vi "PPS Persistent TCP parser server.vi"(8 "error in":errorcluster, 9 "TCP queue name":string="parser_error", 10 "Ignore errors":bool=TRUE, 11 "port":u16=2056) -> (0 "error out":errorcluster)   [LabVIEW 2016]
uses:
  <vilib>/Utility/error.llb/DialogType.ctl
  <vilib>/Utility/error.llb/whitespace.ctl
panel:
  out "Listening":bool=TRUE
  out "Control labels":string
  out "Explanation":string
  out "created new?":bool
  out "TCP error queue":refnum<queue>
  out "cycle msec":u32
  out "Cmd Rec'd":bool
  out "Calling VI's Controls":string[](array[string])
  out "Idle loop":i32
  out "Heartbeat":bool=TRUE
  in  "bytes to read":i32=256
  out "ack":string
  in  "stop":bool=TRUE
  # "This subVI is currently written to handle controls of numeric (\"Digital\", \"Numeric\", \"Ring\"), string and boolean types, and queries of simple clusters and boolean & numeric arrays."
  # "# Example Python program\n\n# Drop this subVI into the VI you want to remote-enable.\n\n#  Here we assume the remote VI has an indicator named \"DisplayValue\" and a control named \"NumberControl\",\n#  and that an event is driven by a value change for NumberControl.\n\nimport os\nimport socket\nimport time\n\nTCP_IP = '127.0.0.1'  #...for VI running on same machine.  Else put IP address of remote machine.\nTCP_PORT = 2056  # Set the port in the VI that calls the parser server.  \nBUFFER_SIZE = 1024\n\n\n\ndef Transact(Command, IsAQuery):   \n\n    StuffToSend = Command + '\\r' + '\\n'   # The TCP Parser Server is looking for cr-lf termination\n    s.send(StuffToSend)\n    response = s.recv(BUFFER_SIZE)   # Communications is much more reliable if you read the response.  \n                                                               # Ideally, compare it to what you sent.  For simplicity we are not doing that here.\n\n    if IsAQuery:\n        response = response.translate(None,'\\r''\\n')  #remove terminator characters\n        return response\n\n#====== Here's the program =====\n\nprint 'Opening socket'\n\ns = socket.socket(socket.AF_INET, socket.SOCK_STREAM)\ns.setsockopt(socket.SOL_SOCKET, socket.SO_REUSEADDR, 1)\ns.connect((TCP_IP, TCP_PORT))\n\n\nfor i in range (1,5000):\n    QueryString = 'DisplayValue?'\n    CommandString = 'NumberControl=' + str(i)\n\n# Send a command\n    Transact (CommandString, False) # False indicates it is not a query\n\n# Perform a query and display the response\n    print 'Received:' + (Transact(QueryString, True)) # 'True' indicates it is a query\n    \n    \n    \ns.shutdown(socket.SHUT_RDWR)\ntime.sleep(0.02) # Delay to prevent a possible Windows error.  20msec is very generous.\ns.close()"
  # "This VI listens on the specified TCP port until a terminated command or query is seen.\n\n-- Command format: \"[Control name] = [new value] [CR][LF]\n\nThis VI will always echo the command it receives (after a CR/LF termination) in the ack indicator, also with CR/LF termination.  Good practice is to compare this return with the issued command to ensure against error.\n\n\n-- Query format: \"[Control or indicator name]?[CR][LF]\"  \n\nAfter query, the ack indicator will contain [Control or indicator name]=[value][CR][LF] \n\nWhite space in commands/queries is ignored.  Control names are case sensitive.\n\nSeparate array elements with tab characters, e.g.; NumberArray = 1\\t2\\t3\\t[CR][LF]\nSeparate cluster elements with vertical-bar characters, e.g.; error out|status?[CR][LF]"
  # "This parser can be made re-entrant to allow scripting of >1 top-level VIs.  The port is set by the calling VI,  take care not to duplicate.\n\nThe calling VI's front-panel controls are available in the indicator to the right.  Since this VI will not return until terminated, read the Calling VI's Controls indicator using a VI reference.  \n\nThe calling VI should have an Event Structure that fires on value change of the controls you want to remote-enable.   Currently supported types are Boolean, Digital (numeric) and String. \n\nAny front-panel control of a supported type can be queried.  \n\nThe instantaneous error status of this VI is available in a named queue.  The name is provided by the calling VI and must be unique.  (The name of the calling VI is a good choice.)"
  # "Note: we trap and internally handle error 66, which indicates a connection was closed.  \nWhen this occurs we simply re-open the connection.\nThis allows a remote host to run and finish many times."
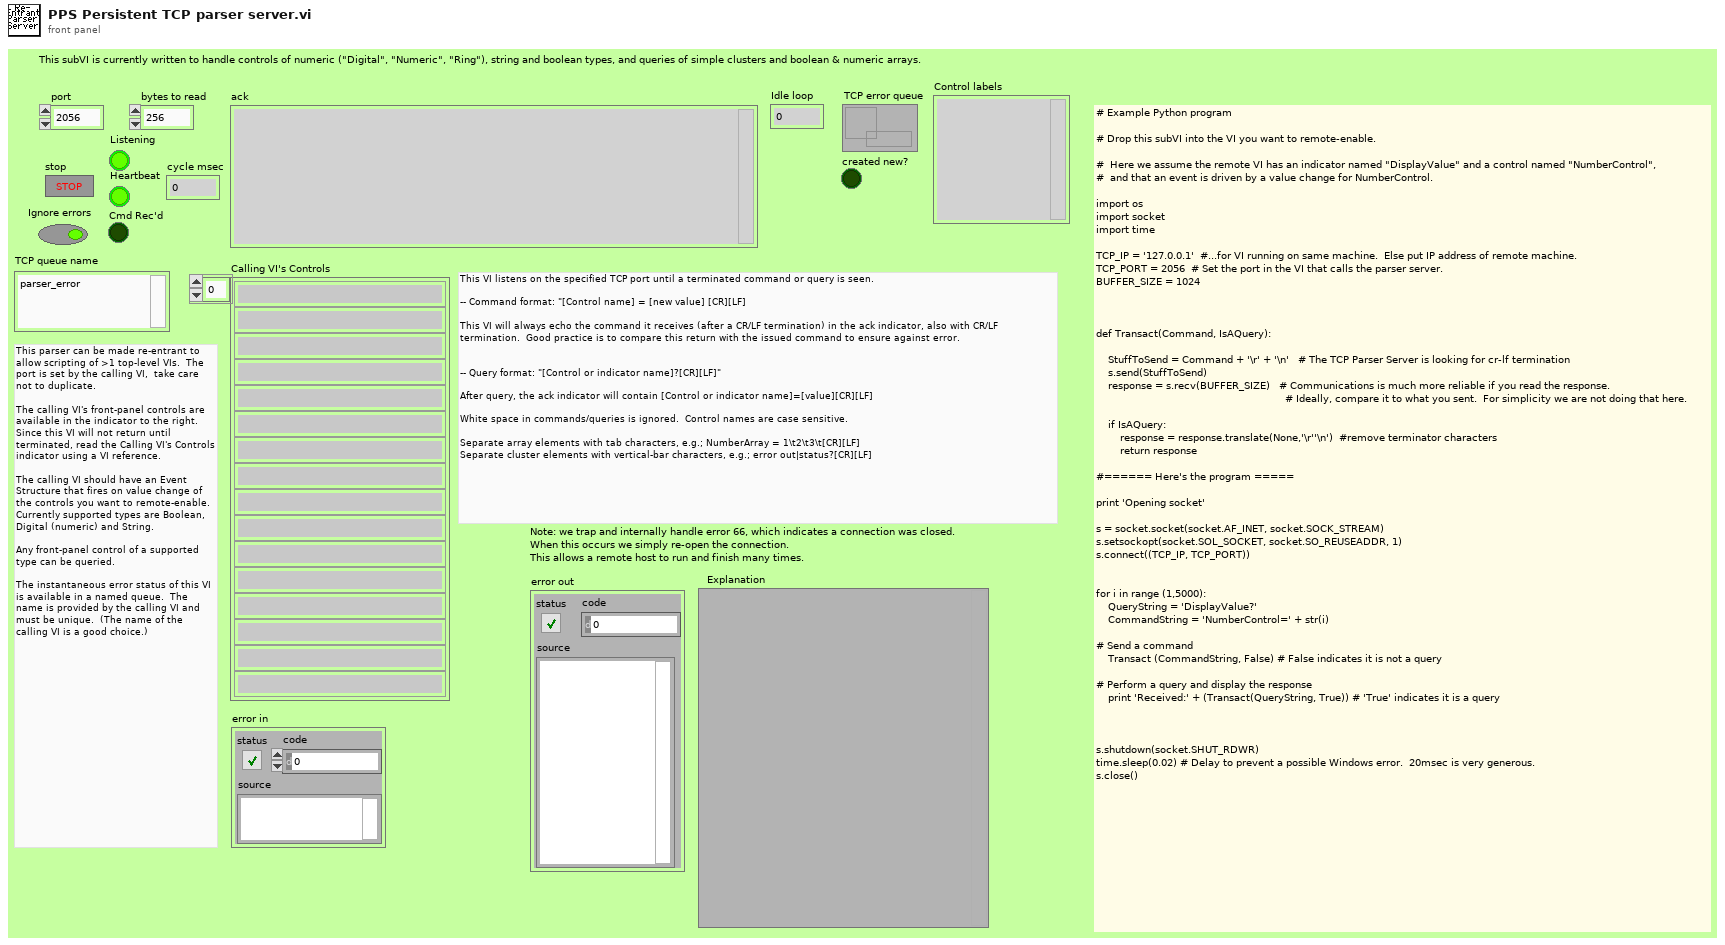
[diagram p1: front panel]
types:
  T1 = enum16{"Standard", "Buffered", "CRLF", "Immediate"}
  T2 = typedef "DialogType.ctl" = u16
  T3 = typedef "whitespace.ctl" = u16
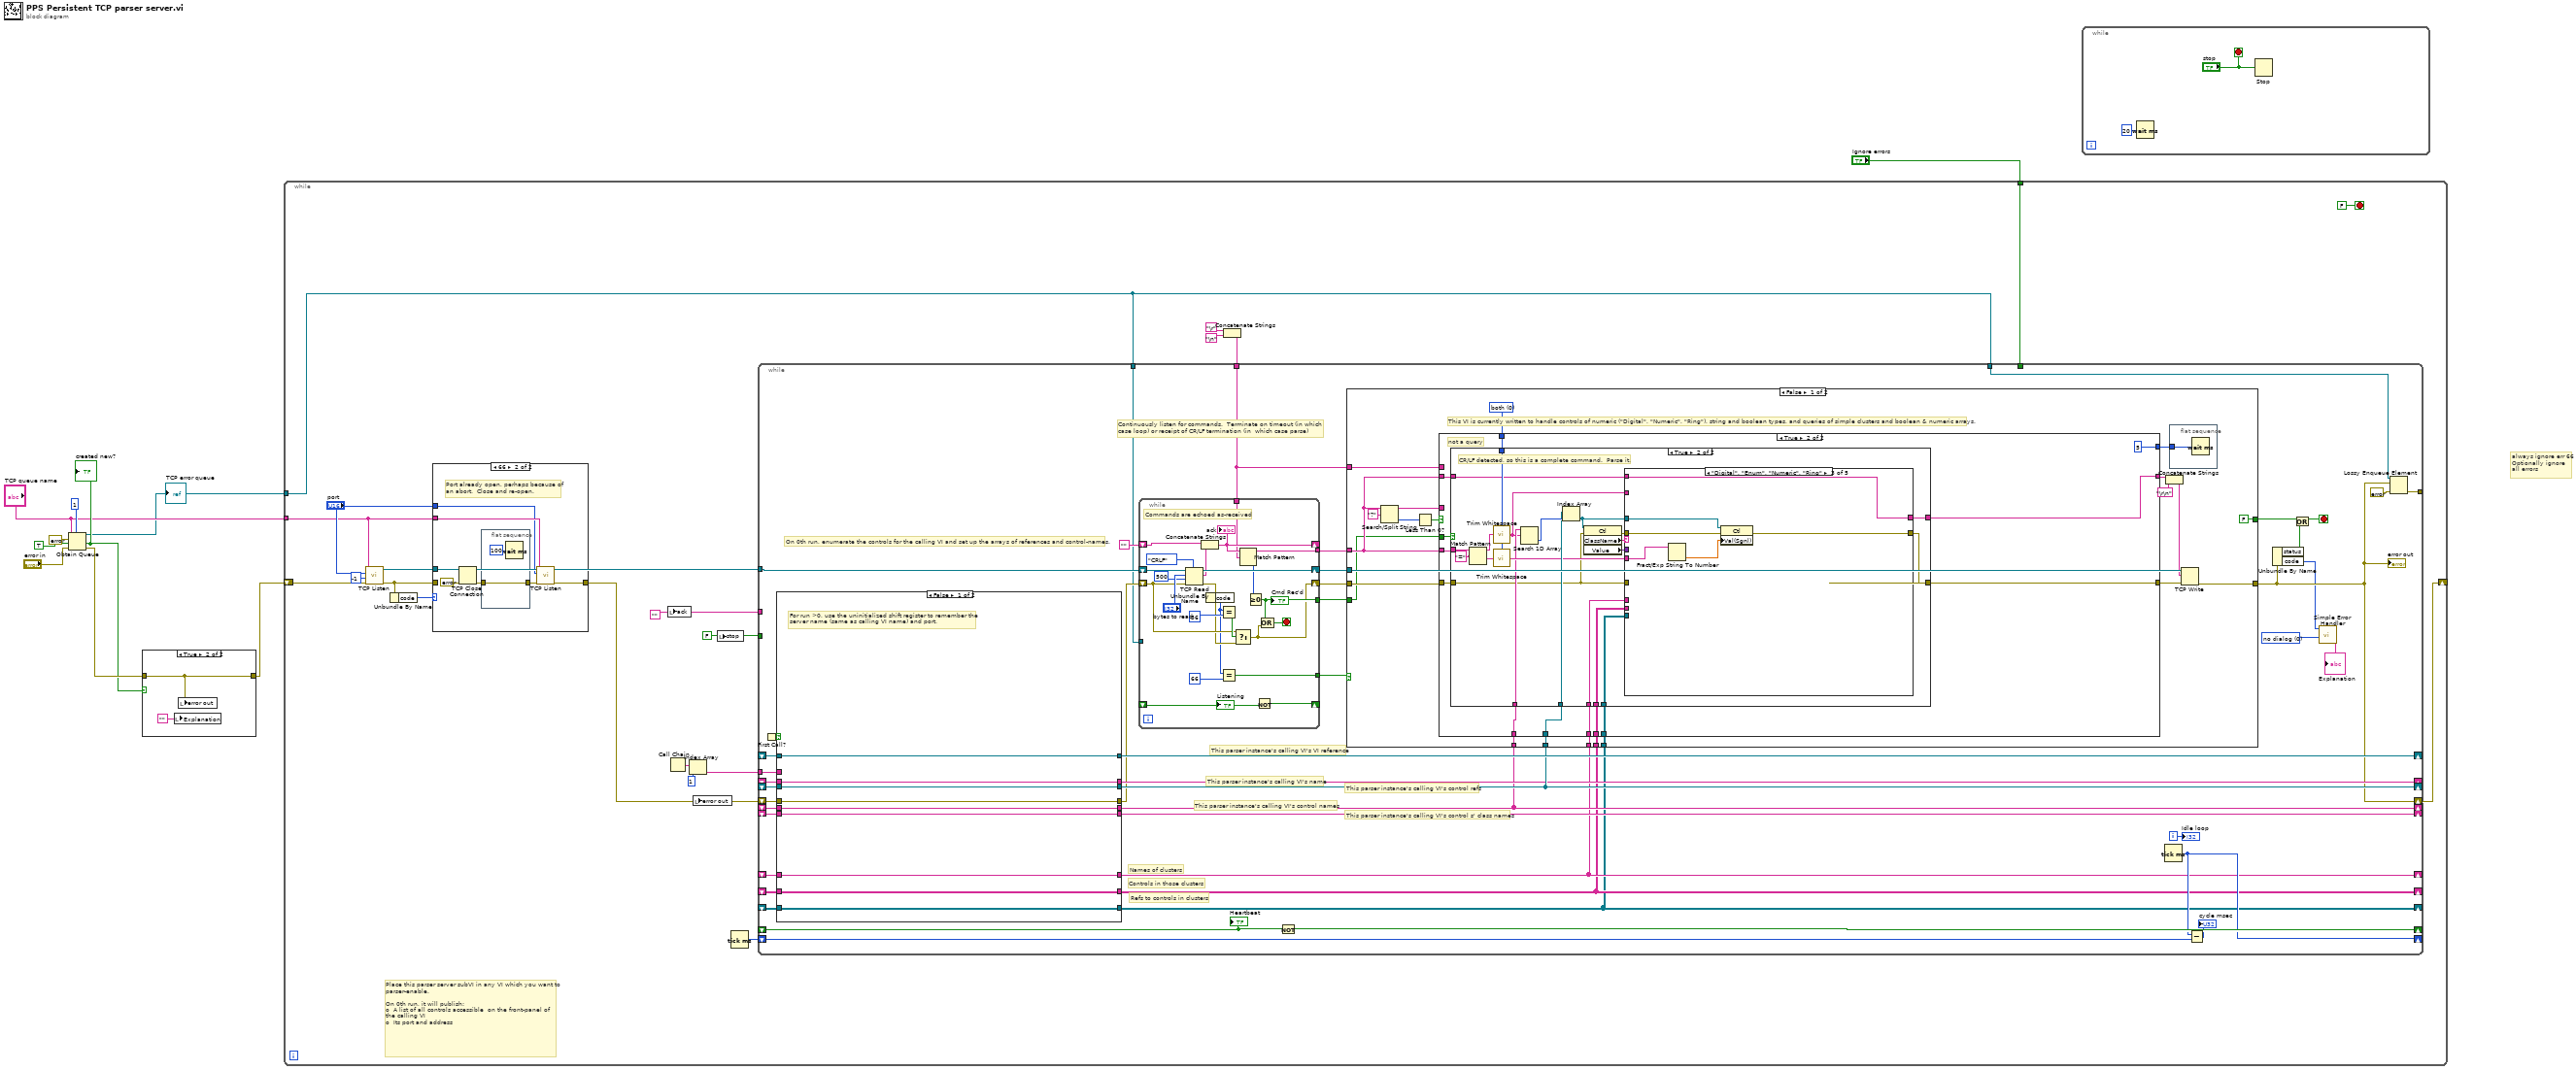
[diagram p0: block diagram]
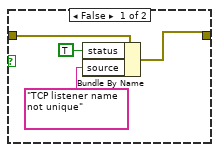
[diagram p2: hidden frame]
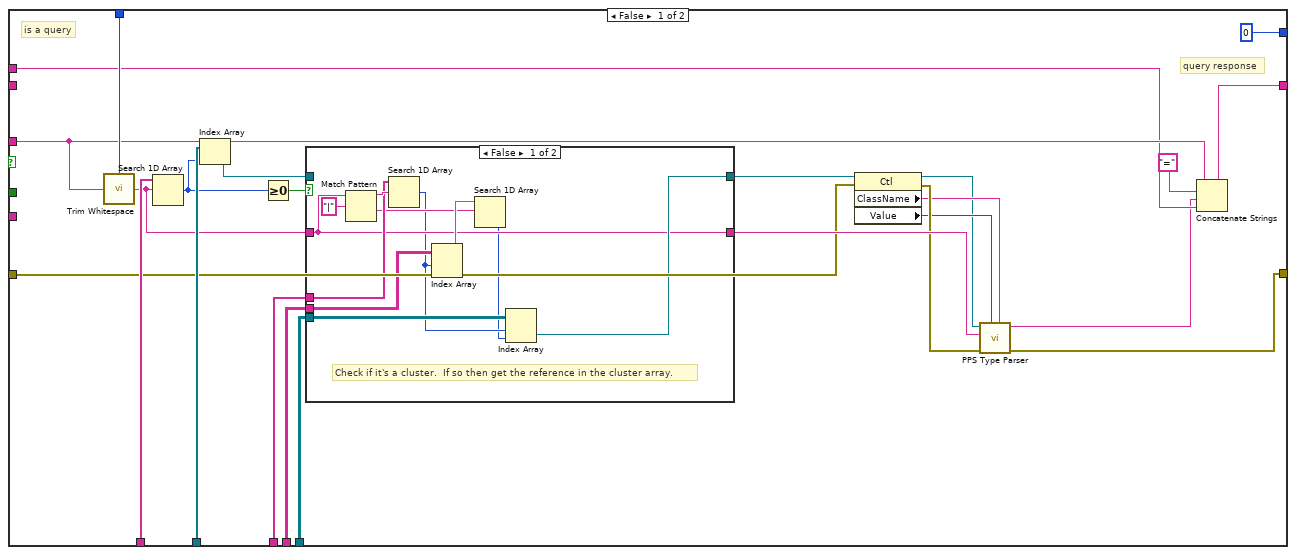
[diagram p4: hidden frame]
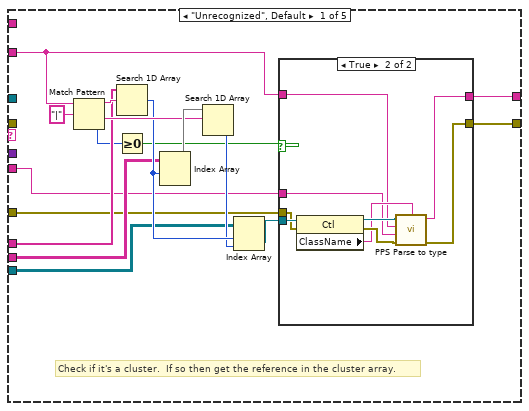
[diagram p7: hidden frame]
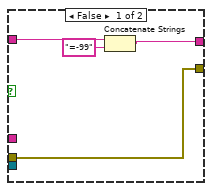
[diagram p8: hidden frame]
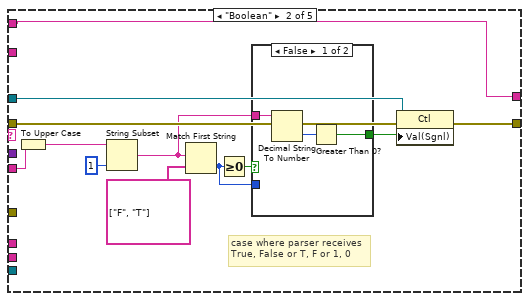
[diagram p9: hidden frame]
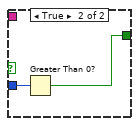
[diagram p10: hidden frame]
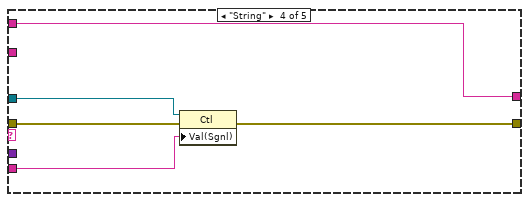
[diagram p11: hidden frame]
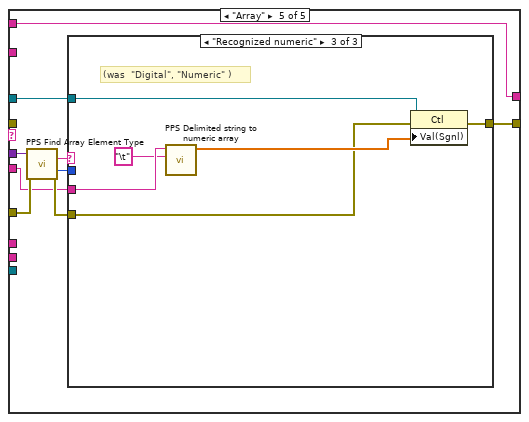
[diagram p12: hidden frame]
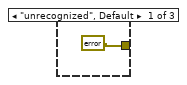
[diagram p13: hidden frame]
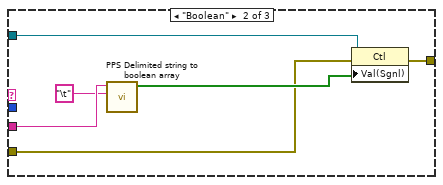
[diagram p14: hidden frame]
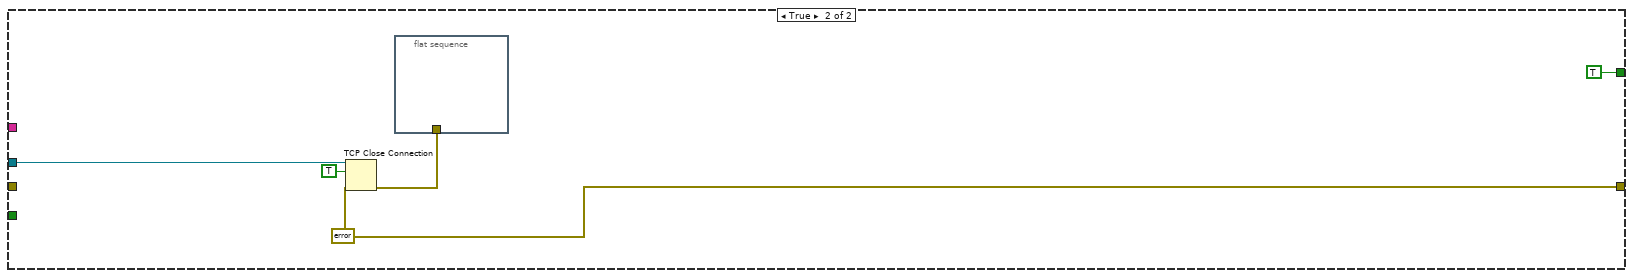
[diagram p15: hidden frame]
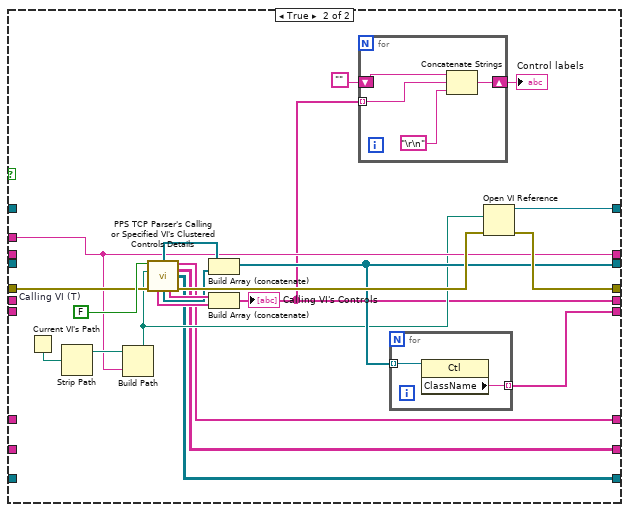
[diagram p16: hidden frame]
diagram:
  # "always ignore err 66\nOptionally ignore\nall errors"
  n1 = Obtain Queue(max queue size (-1, unlimited)=1, name (unnamed)="TCP queue name", element data type=errorcluster {"status"=FALSE, "code"=0, "source"=""} ("error out"), create if not found? (T)=TRUE, error in (no error)="error in") -> (queue out=w3:refnum<queue>, created new?=w9:bool, error out=w10:errorcluster)
  "TCP error queue" <- w3
  "created new?" <- w9
  n2 = case shown="True" w9 {
    tunnel: w10 -> [w14 w16]
    tunnel: [w11 w16] -> w2
    frame False {
      n3 = Bundle By Name(cluster=w14, "status"=TRUE, "source"="TCP listener name not unique") -> (w11:errorcluster)
    }
    frame True {
      n4 = local write "Explanation"("") -> ()
      n5 = local write "error out"(w16) -> ()
    }
  }
  n6 = while {
    tunnel: "TCP queue name" -> [w24]
    tunnel: w3 -> [w21]
    tunnel: "Ignore errors" -> [w19]
    shift-right: [w18] -> _
    shift-left: w2 -> [w23]
    stop <- FALSE stop-if-true
    w33 = ""
    w34 = FALSE ("stop")
    # "Place this parser server subVI in any VI which you want to\nparser-enable.  \n\nOn 0th run, it will publish:\no  A list of all controls accessible  on the front-panel of \nthe calling VI\no  Its port and address"
    n7 = call <vilib>:"TCP Listen.vi"("error in (no error)"=w23, "timeout ms (wait forever: -1)"=-1, "port"="port", "service name"=w24) -> ("error out"=w27:errorcluster, "connection ID"=w20:refnum<k5>)  [unwired: 3 in, 3 out]
    n8 = Unbundle By Name(w27) -> ("code"=w28:i32)
    n9 = case shown="66" w28 {
      tunnel: w27 -> [w38 _]
      tunnel: [w38 w44] -> w25
      tunnel: w20 -> [_ w45]
      tunnel: w24 -> [_ w43]
      tunnel: "port" -> [_ w41]
      frame 0, Default {
      }
      frame 66 {
        # "Port already open, perhaps because of\nan abort.  Close and re-open."
        n10 = TCP Close Connection(connection ID=w45, error in (no error)=errorcluster {"status"=FALSE, "code"=0, "source"=""}) -> (error out=w42:errorcluster)  [unwired: 1 in, 1 out]
        n11 = flat-sequence {
          tunnel: [w46] -> w40
          tunnel: w42 -> [w46]
          frame #0 {
            n12 = Wait (ms)(milliseconds to wait=u32 100) -> ()  [unwired: 1 out]
          }
        }
        n13 = call <vilib>:"TCP Listen.vi"("error in (no error)"=w40, "port"=w41, "service name"=w43) -> ("error out"=w44:errorcluster)  [unwired: 4 in, 4 out]
      }
    }
    n14 = local write "ack"(w33) -> ()
    n15 = Call Chain() -> (call chain=w32:string[])
    n16 = Index Array(array=w32, index=1) -> (element=w30:string)
    n17 = local write "error out"(w25) -> ()
    n18 = local write "stop"(w34) -> ()
    n19 = Tick Count (ms)() -> (millisecond timer value=w29:u32)
    n20 = Concatenate Strings("\r", "\n") -> (w35:string)
    n21 = while {
      tunnel: w34 -> [_]
      shift-right: [w91] -> _
      shift-left: _ -> [w92]
      shift-right: [w80] -> _
      shift-left: _ -> [w89]
      shift-right: [w52] -> w18
      shift-left: w25 -> [w88]
      shift-right: [w87] -> _
      shift-left: _ -> [w86]
      tunnel: w35 -> [w68]
      shift-right: [w84] -> _
      shift-left: _ -> [w85]
      tunnel: w33 -> [_]
      shift-right: [w82] -> _
      shift-left: _ -> [w83]
      tunnel: w30 -> [w81]
      shift-right: [w78] -> _
      shift-left: w29 -> [w77]
      tunnel: w21 -> [w58]
      tunnel: w20 -> [w73]
      shift-right: [w71] -> _
      shift-left: _ -> [w70]
      tunnel: w21 -> [w65]
      shift-right: [w61] -> _
      shift-left: _ -> [w64]
      shift-right: [w60] -> _
      shift-left: _ -> [w63]
      shift-right: [w59] -> _
      shift-left: _ -> [w62]
      tunnel: w19 -> [_]
      tunnel: [w57] -> _
      i -> [w90]
      stop <- w50 stop-if-true
      w53 = T2 0 items=["no dialog", "OK message", "continue or stop message", "OK message + warnings", "continue/stop + warnings"] ("type of dialog (OK msg:1)")
      # "Refs to controls in clusters"
      # "Controls in those clusters"
      # "Names of clusters"
      # "This parser instance's calling VI's control names"
      # "This parser instance's calling VI's control s' class names"
      # "Continuously listen for commands.  Terminate on timeout (in which \ncase loop) or receipt of CR/LF termination (in  which case parse)"
      # "On 0th run, enumerate the controls for the calling VI and set up the arrays of references and control-names."
      # "This parser instance's calling VI's control refs"
      # "This parser instance's calling VI's VI reference"
      # "This parser instance's calling VI's name"
      n22 = First Call?() -> (First Call?: T/F=w79:bool)
      n23 = case shown="False" w79 {
        tunnel: [w305 w313] -> w80
        tunnel: w89 -> [w305 _]
        tunnel: w88 -> [w304 w323]
        tunnel: [w304 w320] -> w72
        tunnel: [w303 w321] -> w87
        tunnel: w86 -> [w303 _]
        tunnel: [w302 w315] -> w84
        tunnel: w85 -> [w302 _]
        tunnel: [w301 w314] -> w82
        tunnel: w83 -> [w301 _]
        tunnel: w81 -> [_ w313]
        tunnel: [w300 w311] -> w71
        tunnel: w70 -> [w300 _]
        tunnel: [w299 w309] -> w61
        tunnel: [w298 w308] -> w60
        tunnel: [w297 w307] -> w59
        tunnel: w64 -> [w299 _]
        tunnel: w63 -> [w298 _]
        tunnel: w62 -> [w297 _]
        frame False {
          # "For run >0, use the uninitialized shift register to remember the \nserver name (same as calling VI name) and port."
        }
        frame True {
          w324 = FALSE  # Calling VI (T)
          n24 = Current VI's Path() -> (path=w316:path)
          n25 = Strip Path(path=w316) -> (stripped path=w317:path)  [unwired: 1 out]
          n26 = Build Path(base path=w317, name or relative path=w313) -> (appended path=w312:path)
          n27 = call "PPS TCP Parser's Calling or Specified VI's Clustered Controls Details.vi"("Calling VI (T)"=w324, "Specified VI (if Calling VI = F)"=w312, "error in (no error)"=w323) -> ("Refs to controls on panel"=w318:refnum<vi>[], "Names of Clusters"=w309:string[], "Controls in\nthose clusters"=w308:string[][], "Refs to controls in clusters"=w307:refnum<vi>[][], "Controls directly on tab panes"=w326:string[], "Refs to controls directly on tab panes"=w319:refnum<vi>[], "Controls on panel"=w325:string[], "error out"=w322:errorcluster)  [unwired: 2 in, 3 out]
          n28 = Build Array (concatenate)(w318, w319) -> (w315:refnum<vi>[])
          n29 = Build Array (concatenate)(w325, w326) -> (w311:string[])
          "Calling VI's Controls" <- w311
          n30 = for {
            shift-right: [w330] -> w310
            shift-left: "" -> [w329]
            tunnel: w311 -> [w327] mode=indexing
            n31 = Concatenate Strings(w329, w327, "\r\n") -> (w330:string)
          }
          "Control labels" <- w310
          n32 = for {
            tunnel: w315 -> [w332] mode=indexing
            tunnel: [w331] -> w314 mode=indexing
            n33 = property class="Ctl"(reference=w332) -> ("ClassName"=w331:string)  [unwired: 1 in, 2 out]
          }
          n34 = Open VI Reference(vi path=w312, error in (no error)=w322) -> (vi reference=w321:refnum<vi>, error out=w320:errorcluster)  [unwired: 4 in]
        }
      }
      n35 = while {
        shift-right: [w293] -> w74
        shift-left: w73 -> [w292]
        shift-right: [w279] -> w75
        shift-left: w72 -> [w281]
        shift-right: [w289] -> _
        shift-left: "" -> [w291]
        tunnel: w68 -> [w288]
        tunnel: [w286] -> w67
        tunnel: [w284] -> w66
        tunnel: w65 -> [_]
        tunnel: [w276] -> w55
        shift-right: [w275] -> _
        shift-left: _ -> [w274]
        stop <- w285 stop-if-true
        # "Commands are echoed as-received"
        n36 = TCP Read(connection ID=w292, bytes to read="bytes to read", error in (no error)=w281, 7:T1."CRLF" ("mode (standard)"), 9:500 ("timeout ms (25000)")) -> (connection ID out=w293:refnum<k5>, data out=w290:string, error out=w280:errorcluster)
        n37 = Concatenate Strings(w291, w290) -> (w289:string)
        "ack" <- w289
        n38 = Unbundle By Name(w280) -> ("code"=w278:i32)
        n39 = Equal?(x=w278, y=56 ("code")) -> (x = y?=w282:bool)
        n40 = Equal?(x=w278, y=66 ("code")) -> (x = y?=w276:bool)
        n41 = Select(t=w281, s=w282, f=w280) -> (s? t:f=w279:errorcluster)
        n42 = Match Pattern(string=w289, regular expression=w288) -> (before substring=w286:string, offset past match=w287:i32)  [unwired: 1 in, 2 out]
        n43 = Greater Or Equal To 0?(x=w287) -> (x >= 0?=w284:bool)
        "Cmd Rec'd" <- w284
        n44 = Not(x=w274) -> (.not. x?=w275:bool)
        n45 = Compound Arithmetic op=OR(w284, w279) -> (w285:bool)
        "Listening" <- w274
      }
      n46 = Not(x=w92) -> (.not. x?=w91:bool)
      n47 = case shown="False" w55 {
        tunnel: w84 -> [w114 _]
        tunnel: w75 -> [w112 _]
        tunnel: w74 -> [w107 w272]
        tunnel: w71 -> [w106 _]
        tunnel: w68 -> [w105 _]
        tunnel: w67 -> [w104 _]
        tunnel: w66 -> [w103 _]
        tunnel: w61 -> [w98 _]
        tunnel: w60 -> [w97 _]
        tunnel: w59 -> [w96 _]
        tunnel: [w94 w270] -> w52
        tunnel: [FALSE TRUE] -> w48
        frame False {
          w108 = T3 0 items=["both", "start of string", "end of string"] ("location (both)")
          # "This VI is currently written to handle controls of numeric (\"Digital\", \"Numeric\", \"Ring\"), string and boolean types, and queries of simple clusters and boolean & numeric arrays."
          n48 = Search/Split String(string=w104, search string/char (-)="?") -> (substring before match=w109:string, offset of match=w110:i32)  [unwired: 1 in, 1 out]
          n49 = Less Than 0?(x=w110) -> (x < 0?=w111:bool)
          n50 = case shown="True" w111 {
            tunnel: w114 -> [w138 w165]
            tunnel: w104 -> [_ w164]
            tunnel: w103 -> [_ w163]
            tunnel: w112 -> [w116 w162]
            tunnel: [w133 w161] -> w95
            tunnel: w109 -> [w137 _]
            tunnel: w108 -> [w139 w160]
            tunnel: w105 -> [w135 _]
            tunnel: w104 -> [_ w153]
            tunnel: [w134 w154] -> w102
            tunnel: w106 -> [w130 w159]
            tunnel: [u32 0 ("milliseconds to wait") u32 5 ("milliseconds to wait")] -> w99
            tunnel: w98 -> [w124 w157]
            tunnel: w97 -> [w123 w156]
            tunnel: w96 -> [w122 w155]
            frame False {
              # "query response"
              # "is a query"
              n51 = call <vilib>:"Trim Whitespace.vi"("string"=w137, "location (both)"=w139) -> ("trimmed string"=w126:string)
              n52 = Search 1D Array(1D array=w130, element=w126) -> (index of element=w128:i32)  [unwired: 1 in]
              n53 = Index Array(array=w138, index=w128) -> (element=w132:refnum<vi>)
              n54 = Greater Or Equal To 0?(x=w128) -> (x >= 0?=w127:bool)
              n55 = case shown="False" w127 {
                tunnel: w132 -> [_ w151]
                tunnel: w126 -> [w142 w152]
                tunnel: [w142 w152] -> w125
                tunnel: w124 -> [w148 _]
                tunnel: w123 -> [w147 _]
                tunnel: w122 -> [w144 _]
                tunnel: [w143 w151] -> w121
                frame False {
                  # "Check if it's a cluster.  If so then get the reference in the cluster array."
                  n56 = Match Pattern(string=w142, regular expression="|") -> (before substring=w150:string, after substring=w145:string)  [unwired: 1 in, 2 out]
                  n57 = Search 1D Array(1D array=w148, element=w150) -> (index of element=w141:i32)  [unwired: 1 in]
                  n58 = Index Array(array=w147, index (row)=w141) -> (element=w146:string[])  [unwired: 1 in]
                  n59 = Search 1D Array(1D array=w146, element=w145) -> (index of element=w140:i32)  [unwired: 1 in]
                  n60 = Index Array(array=w144, index (row)=w141, index (col)=w140) -> (element=w143:refnum<vi>)
                }
                frame True {
                }
              }
              n61 = property class="Ctl"(reference=w121, error in=w116) -> (reference out=w117:refnum<vi>, error out=w120:errorcluster, "ClassName"=w119:string, "Value"=w118:variant)
              n62 = call "PPS Type Parser.vi"("ClassName"=w119, "Value"=w118, "error in (no error)"=w120, "trimmed string"=w125, "Control in"=w117) -> ("error out"=w133:errorcluster, "spreadsheet string"=w131:string)  [unwired: 5 in]
              n63 = Concatenate Strings(w137, "=", w131, w135) -> (w134:string)
            }
            frame True {
              # "not a query"
              n64 = case shown="True" w163 {
                tunnel: w164 -> [_ w188]
                tunnel: w165 -> [_ w183]
                tunnel: [w167 w178] -> w161
                tunnel: w162 -> [w167 w175]
                tunnel: w160 -> [_ w177]
                tunnel: w159 -> [_ w176]
                tunnel: w157 -> [_ w173]
                tunnel: w156 -> [_ w172]
                tunnel: w155 -> [_ w171]
                tunnel: [w166 w169] -> w154
                tunnel: w153 -> [w166 w168]
                frame False {
                  # "CR/LF not found, so this is not a complete command.  Loop."
                }
                frame True {
                  # "CR/LF detected, so this is a complete command.  Parse it."
                  n65 = Match Pattern(string=w188, regular expression="=") -> (before substring=w186:string, after substring=w185:string)  [unwired: 1 in, 2 out]
                  n66 = call <vilib>:"Trim Whitespace.vi"("string"=w186, "location (both)"=w177) -> ("trimmed string"=w170:string)
                  n67 = call <vilib>:"Trim Whitespace.vi"("string"=w185, "location (both)"=w177) -> ("trimmed string"=w181:string)
                  n68 = Search 1D Array(1D array=w176, element=w170) -> (index of element=w184:i32)  [unwired: 1 in]
                  n69 = Index Array(array=w183, index=w184) -> (element=w180:refnum<vi>)
                  n70 = property class="Ctl"(reference=w180, error in=w175) -> (error out=w179:errorcluster, "ClassName"=w182:string, "Value"=w174:variant)  [unwired: 1 out]
                  n71 = case shown="\"Digital\", \"Enum\", \"Numeric\", \"Ring\"" w182 {
                    tunnel: w181 -> [w193 w226 w241 w243 w249]
                    tunnel: w180 -> [_ w229 w240 w246 w248]
                    tunnel: w179 -> [_ w227 w239 w245 _]
                    tunnel: [w192 w230 w238 w244 w255] -> w178
                    tunnel: w175 -> [w190 _ _ _ w253]
                    tunnel: w174 -> [_ _ _ _ w254]
                    tunnel: w173 -> [w199 _ _ _ _]
                    tunnel: w172 -> [w198 _ _ _ _]
                    tunnel: w171 -> [w197 _ _ _ _]
                    tunnel: w170 -> [w189 _ _ _ _]
                    tunnel: [w191 w219 w236 w242 w247] -> w169
                    tunnel: w168 -> [_ w219 w236 w242 w247]
                    frame "Unrecognized", Default {
                      # "Check if it's a cluster.  If so then get the reference in the cluster array."
                      n72 = Match Pattern(string=w189, regular expression="|") -> (before substring=w205:string, after substring=w202:string, offset past match=w196:i32)  [unwired: 1 in, 1 out]
                      n73 = Search 1D Array(1D array=w199, element=w205) -> (index of element=w201:i32)  [unwired: 1 in]
                      n74 = Greater Or Equal To 0?(x=w196) -> (x >= 0?=w195:bool)
                      n75 = Index Array(array=w198, index (row)=w201) -> (element=w203:string[])  [unwired: 1 in]
                      n76 = Search 1D Array(1D array=w203, element=w202) -> (index of element=w200:i32)  [unwired: 1 in]
                      n77 = Index Array(array=w197, index (row)=w201, index (col)=w200) -> (element=w194:refnum<vi>)
                      n78 = case shown="True" w195 {
                        tunnel: w194 -> [_ w218]
                        tunnel: w193 -> [_ w210]
                        tunnel: [w209 w215] -> w192
                        tunnel: [w206 w214] -> w191
                        tunnel: w190 -> [w209 w213]
                        tunnel: w189 -> [w208 w211]
                        frame False {
                          n79 = Concatenate Strings(w208, "=-99" ("string")) -> (w206:string)
                        }
                        frame True {
                          n80 = property class="Ctl"(reference=w218, error in=w213) -> (reference out=w217:refnum<vi>, error out=w216:errorcluster, "ClassName"=w212:string)
                          n81 = call "PPS Parse to type.vi"("ClassName"=w212, "error in (no error)"=w216, "User's new value"=w210, "Control name"=w211, "Control in"=w217) -> ("error out"=w215:errorcluster, "ack"=w214:string)  [unwired: 5 in]
                        }
                      }
                    }
                    frame "Boolean" {
                      # "case where parser receives\nTrue, False or T, F or 1, 0"
                      n82 = To Upper Case(1:w226) -> (0:w222:string)
                      n83 = String Subset(string=w222, length (rest)=1 ("length (rest)")) -> (substring=w220:string)  [unwired: 1 in]
                      n84 = Match First String(2:string[] ["F", "T"] ("string array"), 3:w220) -> (0:w223:i32)  [unwired: 1 out]
                      n85 = Greater Or Equal To 0?(x=w223) -> (x >= 0?=w224:bool)
                      n86 = case shown="False" w224 {
                        tunnel: w223 -> [_ w235]
                        tunnel: w220 -> [w232 _]
                        tunnel: [w231 w234] -> w228
                        frame False {
                          n87 = Decimal String To Number(string=w232) -> (number=w233:i32)  [unwired: 2 in, 1 out]
                          n88 = Greater Than 0?(x=w233) -> (x > 0?=w231:bool)
                        }
                        frame True {
                          n89 = Greater Than 0?(x=w235) -> (x > 0?=w234:bool)
                        }
                      }
                      n90 = property class="Ctl"(reference=w229, error in=w227, "Val(Sgnl)"=w228) -> (error out=w230:errorcluster)  [unwired: 1 out]
                    }
                    frame "Digital", "Enum", "Numeric", "Ring" {
                      n91 = Fract/Exp String To Number(string=w241) -> (number=w237:dbl)  [unwired: 3 in, 1 out]
                      n92 = property class="Ctl"(reference=w240, error in=w239, "Val(Sgnl)"=w237) -> (error out=w238:errorcluster)  [unwired: 1 out]
                    }
                    frame "String" {
                      n93 = property class="Ctl"(reference=w246, error in=w245, "Val(Sgnl)"=w243) -> (error out=w244:errorcluster)  [unwired: 1 out]
                    }
                    frame "Array" {
                      n94 = call "PPS Find Array Element Type.vi"("Variant"=w254, "error in (no error)"=w253) -> ("Element type Name"=w251:string, "Number of Dimensions"=w250:i32, "error out"=w252:errorcluster)  [unwired: 9 in, 2 out]
                      n95 = case shown="\"Recognized numeric\"" w251 {
                        tunnel: [errorcluster {"status"=FALSE, "code"=0, "source"=""} ("error in (no error)") w261 w267] -> w255
                        tunnel: w252 -> [_ w257 w263]
                        tunnel: w250 -> [_ _ _]
                        tunnel: w249 -> [_ w260 w266]
                        tunnel: w248 -> [_ w262 w268]
                        frame "unrecognized", Default {
                        }
                        frame "Boolean" {
                          n96 = call "PPS Delimited string to boolean array.vi"("delimiter"="\t", "1D string of Booleans separated by delimiter"=w260) -> ("Boolean array"=w258:bool[])  [unwired: 9 in]
                          n97 = property class="Ctl"(reference=w262, error in=w257, "Val(Sgnl)"=w258) -> (error out=w261:errorcluster)  [unwired: 1 out]
                        }
                        frame "Recognized numeric" {
                          # "(was  \"Digital\", \"Numeric\" )"
                          n98 = call "PPS Delimited string to numeric array.vi"("delimiter"="\t", "1D string of numerics separated by delimiter"=w266) -> ("Float array"=w264:dbl[])  [unwired: 9 in]
                          n99 = property class="Ctl"(reference=w268, error in=w263, "Val(Sgnl)"=w264) -> (error out=w267:errorcluster)  [unwired: 1 out]
                        }
                      }
                    }
                  }
                }
              }
            }
          }
          n100 = Concatenate Strings(w102, "\r\n") -> (w100:string)
          n101 = flat-sequence {
            tunnel: w99 -> [w115]
            frame #0 {
              n102 = Wait (ms)(milliseconds to wait=w115) -> ()  [unwired: 1 out]
            }
          }
          n103 = TCP Write(connection ID=w107, data in=w100, error in (no error)=w95) -> (error out=w94:errorcluster)  [unwired: 1 in, 2 out]
        }
        frame True {
          w270 = errorcluster {"status"=FALSE, "code"=0, "source"=""} ("error in (no error)")
          n104 = TCP Close Connection(connection ID=w272, abort (F)=TRUE, error in (no error)=w270) -> (error out=w269:errorcluster)  [unwired: 1 out]
          n105 = flat-sequence {
            tunnel: w269 -> [_]
            frame #0 {
            }
          }
        }
      }
      "error out" <- w52
      n106 = Tick Count (ms)() -> (millisecond timer value=w78:u32)
      n107 = Subtract(x=w78, y=w77) -> (x-y=→"cycle msec":u32)
      n108 = Unbundle By Name(w52) -> ("status"=w49:bool, "code"=w51:i32)
      n109 = Or(x=w48, y=w49) -> (x .or. y?=w50:bool)
      n110 = call <vilib>:"Simple Error Handler.vi"("error code (no error:0)"=w51, "type of dialog (OK msg:1)"=w53) -> ("message"=→"Explanation":string)  [unwired: 3 in, 4 out]
      n111 = Lossy Enqueue Element(queue=w58, element=w52, error in (no error)=errorcluster {"status"=FALSE, "code"=0, "source"=""}) -> (error out=w57:errorcluster)  [unwired: 3 out]
      "Heartbeat" <- w92
      "Idle loop" <- w90
    }
  }
  n112 = while {
    stop <- "stop" stop-if-true
    n113 = Wait (ms)(milliseconds to wait=u32 20) -> ()  [unwired: 1 out]
    n114 = Stop(stop? (T)="stop") -> ()
  }
